vi "Experiment header-Interface module.vi"(4 "Value to change":variant, 6 "Name of parameter to update":string, 7 "Header file sections":T21=enum."GLOBAL PARAMETERS", 8 "error in (no error)":errorcluster, 9 "All header parameters in":T1={"LOGIN"={"User"="Olympus  20X", "Profile"="", "Software Version"="", "Experiment Date Time"=timestamp(0 s since 1904-01-01)}, "GLOBAL PARAMETERS"={"MicroscopeID"="", "Microscope Type"="", "Objective"="", "Field of View (um)"=0.0, "Fill time (us)"=0.0, "Experiment Type"=enum."In vivo", "Stimuli Trigger"=FALSE, "Speed Logging"=FALSE}, "IMAGING MODES"={"Time Series"=FALSE, "Motor Zstack"=FALSE, "AOL Zstack"=FALSE, "Functional Imaging"=FALSE, "Volume Imaging"=FALSE}, "TIME SERIES"={"Basic Image meta data"={"Wavelength (nm)"=0.0, "# averaged frames"=0.0, "laser power (%)"=0.0, "Pockels"=0.0, "pixel dwell time (us)"=0.0, "pmt 1"=0.0, "pmt 2"=0.0, "back apperture"=0.0, "zoom"=0.0, "field of view"=0.0, "Frame Size"=0, "AOL x centre"=0.0, "AOL y centre"=0.0, "Stage x position"=0.0, "Stage y position"=0.0, "Stage z position"=0.0}, "AOL z"=0.0}, "MOTOR Z-STACK "={"Hdr Basic Image meta data"={"Wavelength (nm)"=0.0, "# averaged frames"=0.0, "laser power (%)"=0.0, "Pockels"=0.0, "pixel dwell time (us)"=0.0, "pmt 1"=0.0, "pmt 2"=0.0, "back apperture"=0.0, "zoom"=0.0, "field of view"=0.0, "Frame Size"=0, "AOL x centre"=0.0, "AOL y centre"=0.0, "Stage x position"=0.0, "Stage y position"=0.0, "Stage z position"=0.0}, "Z Start"=0.0, "Z Stop"=0.0, "No of Planes"=0, "Laser Power (%) at Z Start"=0.0, "Laser Power (%) at Z Stop"=0.0}, "AOL Z-STACK"={"Hdr Basic Image meta data"={"Wavelength (nm)"=0.0, "# averaged frames"=0.0, "laser power (%)"=0.0, "Pockels"=0.0, "pixel dwell time (us)"=0.0, "pmt 1"=0.0, "pmt 2"=0.0, "back apperture"=0.0, "zoom"=0.0, "field of view"=0.0, "Frame Size"=0, "AOL x centre"=0.0, "AOL y centre"=0.0, "Stage x position"=0.0, "Stage y position"=0.0, "Stage z position"=0.0}, "Z Start"=0.0, "Z Stop"=0.0, "No of Planes"=0, "Laser Power (%) at Z Start"=0.0, "Laser Power (%) at Z Stop"=0.0}, "FUNCTIONAL IMAGING"={"Functional Mode"=enum."Point", "Variable Length"=FALSE, "Variable Resolution"=FALSE, "Pockels Modulation"=FALSE, "Stimuli Trigger"=FALSE, "Cool down enabled"=FALSE, "AOL Mode"=enum."Raster", "Plane Mode"=0, "Miniscan Dwell time per pixel (us)"=0.0, "poi dwell time"=0.0, "Number of trials"=0.0, "Number of cycles"=0.0, "Number of pois"=0.0, "Number of miniscans"=0.0, "Number of pixels in miniscan"=0.0, "Rectangle ROI length"=0.0, "Rectangle ROI height"=0.0, "Frame rate (fps)"=0.0, "Acquisition Length"=0.0, "video length (sec)"=0.0, "Stimuli delay (sec)"=0.0, "Cool down time (sec)"=0.0, "Basic Image meta data"={"Wavelength (nm)"=0.0, "# averaged frames"=0.0, "laser power (%)"=0.0, "Pockels"=0.0, "pixel dwell time (us)"=0.0, "pmt 1"=0.0, "pmt 2"=0.0, "back apperture"=0.0, "zoom"=0.0, "field of view"=0.0, "Frame Size"=0, "AOL x centre"=0.0, "AOL y centre"=0.0, "Stage x position"=0.0, "Stage y position"=0.0, "Stage z position"=0.0}, "Z Start (um)"=0.0, "Z Stop (um)"=0.0}, "VOLUME IMAGING"={"Functional Mode"=enum."Point", "Variable Length"=FALSE, "Variable Resolution"=FALSE, "Pockels Modulation"=FALSE, "Stimuli Trigger"=FALSE, "Cool down enabled"=FALSE, "AOL Mode"=enum."Raster", "Plane Mode"=0, "Miniscan Dwell time per pixel (us)"=0.0, "poi dwell time"=0.0, "Number of trials"=0.0, "Number of cycles"=0.0, "Number of pois"=0.0, "Number of miniscans"=0.0, "Number of pixels in miniscan"=0.0, "Rectangle ROI length"=0.0, "Rectangle ROI height"=0.0, "Frame rate (fps)"=0.0, "Acquisition Length"=0.0, "video length (sec)"=0.0, "Stimuli delay (sec)"=0.0, "Cool down time (sec)"=0.0, "Basic Image meta data"={"Wavelength (nm)"=0.0, "# averaged frames"=0.0, "laser power (%)"=0.0, "Pockels"=0.0, "pixel dwell time (us)"=0.0, "pmt 1"=0.0, "pmt 2"=0.0, "back apperture"=0.0, "zoom"=0.0, "field of view"=0.0, "Frame Size"=0, "AOL x centre"=0.0, "AOL y centre"=0.0, "Stage x position"=0.0, "Stage y position"=0.0, "Stage z position"=0.0}, "Z Start (um)"=0.0, "Z Stop (um)"=0.0}, "MOVEMENT CORRECTION"={"Movement Correction"=FALSE, "Axial Reference"=FALSE, "Reference Source"=enum."Green channel", "Full Frame Size"=0.0, "Reference Field of View"=0.0, "Reference Zoom"=0.0, "Reference dwell time (us)"=0.0, "Reference X Pixels"=0.0, "Reference Y Pixels"=0.0, "Number of Z lines"=0.0, "Size of Z pixels"=0.0, "Axial Pixels"=0.0, "Ignore Z lines"=0.0, "Reference Scan Cycles"=0.0, "Reference Threshold XY"=0.0, "Reference Threshold Z"=0.0, "Reference Average XY"=0.0, "Reference Average Z"=0.0, "Proportional Scale"=0.0, "Integral Scale"=0.0, "Proportional Scale Z"=0.0, "Integral Scale Z"=0.0, "Diff Threshold"=0.0, "Diff Threshold Z"=0.0, "Sliding Average"=FALSE, "Reference count reset enabled"=FALSE, "Scan Interval (ms)"=0.0, "Ref Plot Refresh Rate (ms)"=0.0}, "CALIBRATION"={"Pockels Calibration File"=path "", "Calibration_ini file"=path "", "Setup_ini file"=path ""}, "STATISTICS"={"Z-stack duration (sec)"=0.0, "Number of acquired data-points"=0.0, "Acquisition time (ms)"=0.0, "Number of acquired frames"=0.0, "Intertrial times"=[]}, "BIOLOGY INFORMATION"={"Animal Code or Name"="", "Animal DoB"="", "Animal Age"="", "Animal Sex"="", "Animal Weight"="", "Date of Injection"="", "Date of Implant"="", "Site of Injection"="", "Animal Ear Notch"="", "AAV constructs"="", "Genetic background"="", "Optical reporter"="", "Region of brain imaged"="", "Other \ncomments"=""}, "Calibration Data"={"Objective Name"="", "Calibration Wavelength"=0.0, "Sum X"=0.0, "Sum Y"=0.0, "Diff X"=0.0, "Diff Y"=0.0, "Distortion Correction"=0.0, " Z norm to um Scaling"=0.0, " X norm to um Scaling"=0.0}} {"VOLUME IMAGING"."Plane Mode" items=["XY Plane", "XZ Plane", "YZ Plane", "arbitraryplane"]; "VOLUME IMAGING"."Basic Image meta data"."Frame Size" items=["100X100"=100, "128X128"=128, "200X200"=200, "256X256"=256, "512X512"=512, "1024x1024"=1024, "2048x2048"=2048]; "AOL Z-STACK"."Hdr Basic Image meta data"."Frame Size" items=["100X100"=100, "128X128"=128, "200X200"=200, "256X256"=256, "512X512"=512, "1024x1024"=1024, "2048x2048"=2048]; "MOTOR Z-STACK"."Hdr Basic Image meta data"."Frame Size" items=["100X100"=100, "128X128"=128, "200X200"=200, "256X256"=256, "512X512"=512, "1024x1024"=1024, "2048x2048"=2048]; "FUNCTIONAL IMAGING"."Plane Mode" items=["XY Plane", "XZ Plane", "YZ Plane", "arbitraryplane"]; "FUNCTIONAL IMAGING"."Basic Image meta data"."Frame Size" items=["100X100"=100, "128X128"=128, "200X200"=200, "256X256"=256, "512X512"=512, "1024x1024"=1024, "2048x2048"=2048]; "TIME SERIES"."Basic Image meta data"."Frame Size" items=["100X100"=100, "128X128"=128, "200X200"=200, "256X256"=256, "512X512"=512, "1024x1024"=1024, "2048x2048"=2048]}, 10 "Function":T22, 11 "Experiment data folder path":path) -> (0 "error out":errorcluster, 1 "All params (internal)":T1 {"VOLUME IMAGING"."Plane Mode" items=["XY Plane", "XZ Plane", "YZ Plane", "arbitraryplane"]; "VOLUME IMAGING"."Basic Image meta data"."Frame Size" items=["100X100"=100, "128X128"=128, "200X200"=200, "256X256"=256, "512X512"=512, "1024x1024"=1024, "2048x2048"=2048]; "AOL Z-STACK"."Hdr Basic Image meta data"."Frame Size" items=["100X100"=100, "128X128"=128, "200X200"=200, "256X256"=256, "512X512"=512, "1024x1024"=1024, "2048x2048"=2048]; "MOTOR Z-STACK"."Hdr Basic Image meta data"."Frame Size" items=["100X100"=100, "128X128"=128, "200X200"=200, "256X256"=256, "512X512"=512, "1024x1024"=1024, "2048x2048"=2048]; "FUNCTIONAL IMAGING"."Plane Mode" items=["XY Plane", "XZ Plane", "YZ Plane", "arbitraryplane"]; "FUNCTIONAL IMAGING"."Basic Image meta data"."Frame Size" items=["100X100"=100, "128X128"=128, "200X200"=200, "256X256"=256, "512X512"=512, "1024x1024"=1024, "2048x2048"=2048]; "TIME SERIES"."Basic Image meta data"."Frame Size" items=["100X100"=100, "128X128"=128, "200X200"=200, "256X256"=256, "512X512"=512, "1024x1024"=1024, "2048x2048"=2048]})   [LabVIEW 2020]
uses:
  Typedefs/Header file interface module functions enum.ctl
  Typedefs/Header parameters cluster-ALL.ctl
  Typedefs/Header subclusters/Header params -Login.ctl
  Typedefs/Header subclusters/Header params-Global Parameters.ctl
  Misc/Experiment Type.ctl
  Typedefs/Header subclusters/Header params-Imaging Modes.ctl
  Typedefs/Header subclusters/Header params-Time Series.ctl
  Typedefs/Header subclusters/Header params-Basic image meta data.ctl
  Typedefs/Frame Size.ctl
  Typedefs/Header subclusters/Header params-Motor Z-stack.ctl
  Typedefs/Header subclusters/Header params-AOL Z-stack.ctl
  Typedefs/Header subclusters/Header params-Functional Imaging.ctl
  Typedefs/Functional Mode.ctl
  Typedefs/AOL modes.ctl
  Typedefs/Plane Mode.ctl
  Typedefs/Header subclusters/Header params-Movement correction.ctl
  Typedefs/Reference source.ctl
  Typedefs/Header subclusters/Header params-Calibration Setup.ctl
  Typedefs/Header subclusters/Header params-statistics.ctl
  Misc/Biology Information.ctl
  Typedefs/Header subclusters/Header params-calibration data.ctl
  Typedefs/Header file sections.ctl
  Typedefs/Header file actions.ctl
  Typedefs/Save-Load-Save as-Load last enum.ctl
panel:
  in  "All params (internal)":T1={"LOGIN"={"User"="Olympus  20X", "Profile"="", "Software Version"="", "Experiment Date Time"=timestamp(0 s since 1904-01-01)}, "GLOBAL PARAMETERS"={"MicroscopeID"="", "Microscope Type"="", "Objective"="", "Field of View (um)"=0.0, "Fill time (us)"=0.0, "Experiment Type"=enum."In vivo", "Stimuli Trigger"=FALSE, "Speed Logging"=FALSE}, "IMAGING MODES"={"Time Series"=FALSE, "Motor Zstack"=FALSE, "AOL Zstack"=FALSE, "Functional Imaging"=FALSE, "Volume Imaging"=FALSE}, "TIME SERIES"={"Basic Image meta data"={"Wavelength (nm)"=0.0, "# averaged frames"=0.0, "laser power (%)"=0.0, "Pockels"=0.0, "pixel dwell time (us)"=0.0, "pmt 1"=0.0, "pmt 2"=0.0, "back apperture"=0.0, "zoom"=0.0, "field of view"=0.0, "Frame Size"=0, "AOL x centre"=0.0, "AOL y centre"=0.0, "Stage x position"=0.0, "Stage y position"=0.0, "Stage z position"=0.0}, "AOL z"=0.0}, "MOTOR Z-STACK "={"Hdr Basic Image meta data"={"Wavelength (nm)"=0.0, "# averaged frames"=0.0, "laser power (%)"=0.0, "Pockels"=0.0, "pixel dwell time (us)"=0.0, "pmt 1"=0.0, "pmt 2"=0.0, "back apperture"=0.0, "zoom"=0.0, "field of view"=0.0, "Frame Size"=0, "AOL x centre"=0.0, "AOL y centre"=0.0, "Stage x position"=0.0, "Stage y position"=0.0, "Stage z position"=0.0}, "Z Start"=0.0, "Z Stop"=0.0, "No of Planes"=0, "Laser Power (%) at Z Start"=0.0, "Laser Power (%) at Z Stop"=0.0}, "AOL Z-STACK"={"Hdr Basic Image meta data"={"Wavelength (nm)"=0.0, "# averaged frames"=0.0, "laser power (%)"=0.0, "Pockels"=0.0, "pixel dwell time (us)"=0.0, "pmt 1"=0.0, "pmt 2"=0.0, "back apperture"=0.0, "zoom"=0.0, "field of view"=0.0, "Frame Size"=0, "AOL x centre"=0.0, "AOL y centre"=0.0, "Stage x position"=0.0, "Stage y position"=0.0, "Stage z position"=0.0}, "Z Start"=0.0, "Z Stop"=0.0, "No of Planes"=0, "Laser Power (%) at Z Start"=0.0, "Laser Power (%) at Z Stop"=0.0}, "FUNCTIONAL IMAGING"={"Functional Mode"=enum."Point", "Variable Length"=FALSE, "Variable Resolution"=FALSE, "Pockels Modulation"=FALSE, "Stimuli Trigger"=FALSE, "Cool down enabled"=FALSE, "AOL Mode"=enum."Raster", "Plane Mode"=0, "Miniscan Dwell time per pixel (us)"=0.0, "poi dwell time"=0.0, "Number of trials"=0.0, "Number of cycles"=0.0, "Number of pois"=0.0, "Number of miniscans"=0.0, "Number of pixels in miniscan"=0.0, "Rectangle ROI length"=0.0, "Rectangle ROI height"=0.0, "Frame rate (fps)"=0.0, "Acquisition Length"=0.0, "video length (sec)"=0.0, "Stimuli delay (sec)"=0.0, "Cool down time (sec)"=0.0, "Basic Image meta data"={"Wavelength (nm)"=0.0, "# averaged frames"=0.0, "laser power (%)"=0.0, "Pockels"=0.0, "pixel dwell time (us)"=0.0, "pmt 1"=0.0, "pmt 2"=0.0, "back apperture"=0.0, "zoom"=0.0, "field of view"=0.0, "Frame Size"=0, "AOL x centre"=0.0, "AOL y centre"=0.0, "Stage x position"=0.0, "Stage y position"=0.0, "Stage z position"=0.0}, "Z Start (um)"=0.0, "Z Stop (um)"=0.0}, "VOLUME IMAGING"={"Functional Mode"=enum."Point", "Variable Length"=FALSE, "Variable Resolution"=FALSE, "Pockels Modulation"=FALSE, "Stimuli Trigger"=FALSE, "Cool down enabled"=FALSE, "AOL Mode"=enum."Raster", "Plane Mode"=0, "Miniscan Dwell time per pixel (us)"=0.0, "poi dwell time"=0.0, "Number of trials"=0.0, "Number of cycles"=0.0, "Number of pois"=0.0, "Number of miniscans"=0.0, "Number of pixels in miniscan"=0.0, "Rectangle ROI length"=0.0, "Rectangle ROI height"=0.0, "Frame rate (fps)"=0.0, "Acquisition Length"=0.0, "video length (sec)"=0.0, "Stimuli delay (sec)"=0.0, "Cool down time (sec)"=0.0, "Basic Image meta data"={"Wavelength (nm)"=0.0, "# averaged frames"=0.0, "laser power (%)"=0.0, "Pockels"=0.0, "pixel dwell time (us)"=0.0, "pmt 1"=0.0, "pmt 2"=0.0, "back apperture"=0.0, "zoom"=0.0, "field of view"=0.0, "Frame Size"=0, "AOL x centre"=0.0, "AOL y centre"=0.0, "Stage x position"=0.0, "Stage y position"=0.0, "Stage z position"=0.0}, "Z Start (um)"=0.0, "Z Stop (um)"=0.0}, "MOVEMENT CORRECTION"={"Movement Correction"=FALSE, "Axial Reference"=FALSE, "Reference Source"=enum."Green channel", "Full Frame Size"=0.0, "Reference Field of View"=0.0, "Reference Zoom"=0.0, "Reference dwell time (us)"=0.0, "Reference X Pixels"=0.0, "Reference Y Pixels"=0.0, "Number of Z lines"=0.0, "Size of Z pixels"=0.0, "Axial Pixels"=0.0, "Ignore Z lines"=0.0, "Reference Scan Cycles"=0.0, "Reference Threshold XY"=0.0, "Reference Threshold Z"=0.0, "Reference Average XY"=0.0, "Reference Average Z"=0.0, "Proportional Scale"=0.0, "Integral Scale"=0.0, "Proportional Scale Z"=0.0, "Integral Scale Z"=0.0, "Diff Threshold"=0.0, "Diff Threshold Z"=0.0, "Sliding Average"=FALSE, "Reference count reset enabled"=FALSE, "Scan Interval (ms)"=0.0, "Ref Plot Refresh Rate (ms)"=0.0}, "CALIBRATION"={"Pockels Calibration File"=path "", "Calibration_ini file"=path "", "Setup_ini file"=path ""}, "STATISTICS"={"Z-stack duration (sec)"=0.0, "Number of acquired data-points"=0.0, "Acquisition time (ms)"=0.0, "Number of acquired frames"=0.0, "Intertrial times"=[]}, "BIOLOGY INFORMATION"={"Animal Code or Name"="", "Animal DoB"="", "Animal Age"="", "Animal Sex"="", "Animal Weight"="", "Date of Injection"="", "Date of Implant"="", "Site of Injection"="", "Animal Ear Notch"="", "AAV constructs"="", "Genetic background"="", "Optical reporter"="", "Region of brain imaged"="", "Other \ncomments"=""}, "Calibration Data"={"Objective Name"="", "Calibration Wavelength"=0.0, "Sum X"=0.0, "Sum Y"=0.0, "Diff X"=0.0, "Diff Y"=0.0, "Distortion Correction"=0.0, " Z norm to um Scaling"=0.0, " X norm to um Scaling"=0.0}} {"VOLUME IMAGING"."Plane Mode" items=["XY Plane", "XZ Plane", "YZ Plane", "arbitraryplane"]; "VOLUME IMAGING"."Basic Image meta data"."Frame Size" items=["100X100"=100, "128X128"=128, "200X200"=200, "256X256"=256, "512X512"=512, "1024x1024"=1024, "2048x2048"=2048]; "AOL Z-STACK"."Hdr Basic Image meta data"."Frame Size" items=["100X100"=100, "128X128"=128, "200X200"=200, "256X256"=256, "512X512"=512, "1024x1024"=1024, "2048x2048"=2048]; "MOTOR Z-STACK"."Hdr Basic Image meta data"."Frame Size" items=["100X100"=100, "128X128"=128, "200X200"=200, "256X256"=256, "512X512"=512, "1024x1024"=1024, "2048x2048"=2048]; "FUNCTIONAL IMAGING"."Plane Mode" items=["XY Plane", "XZ Plane", "YZ Plane", "arbitraryplane"]; "FUNCTIONAL IMAGING"."Basic Image meta data"."Frame Size" items=["100X100"=100, "128X128"=128, "200X200"=200, "256X256"=256, "512X512"=512, "1024x1024"=1024, "2048x2048"=2048]; "TIME SERIES"."Basic Image meta data"."Frame Size" items=["100X100"=100, "128X128"=128, "200X200"=200, "256X256"=256, "512X512"=512, "1024x1024"=1024, "2048x2048"=2048]}
  # "Used with the \"Update specific value in memory\" function only"
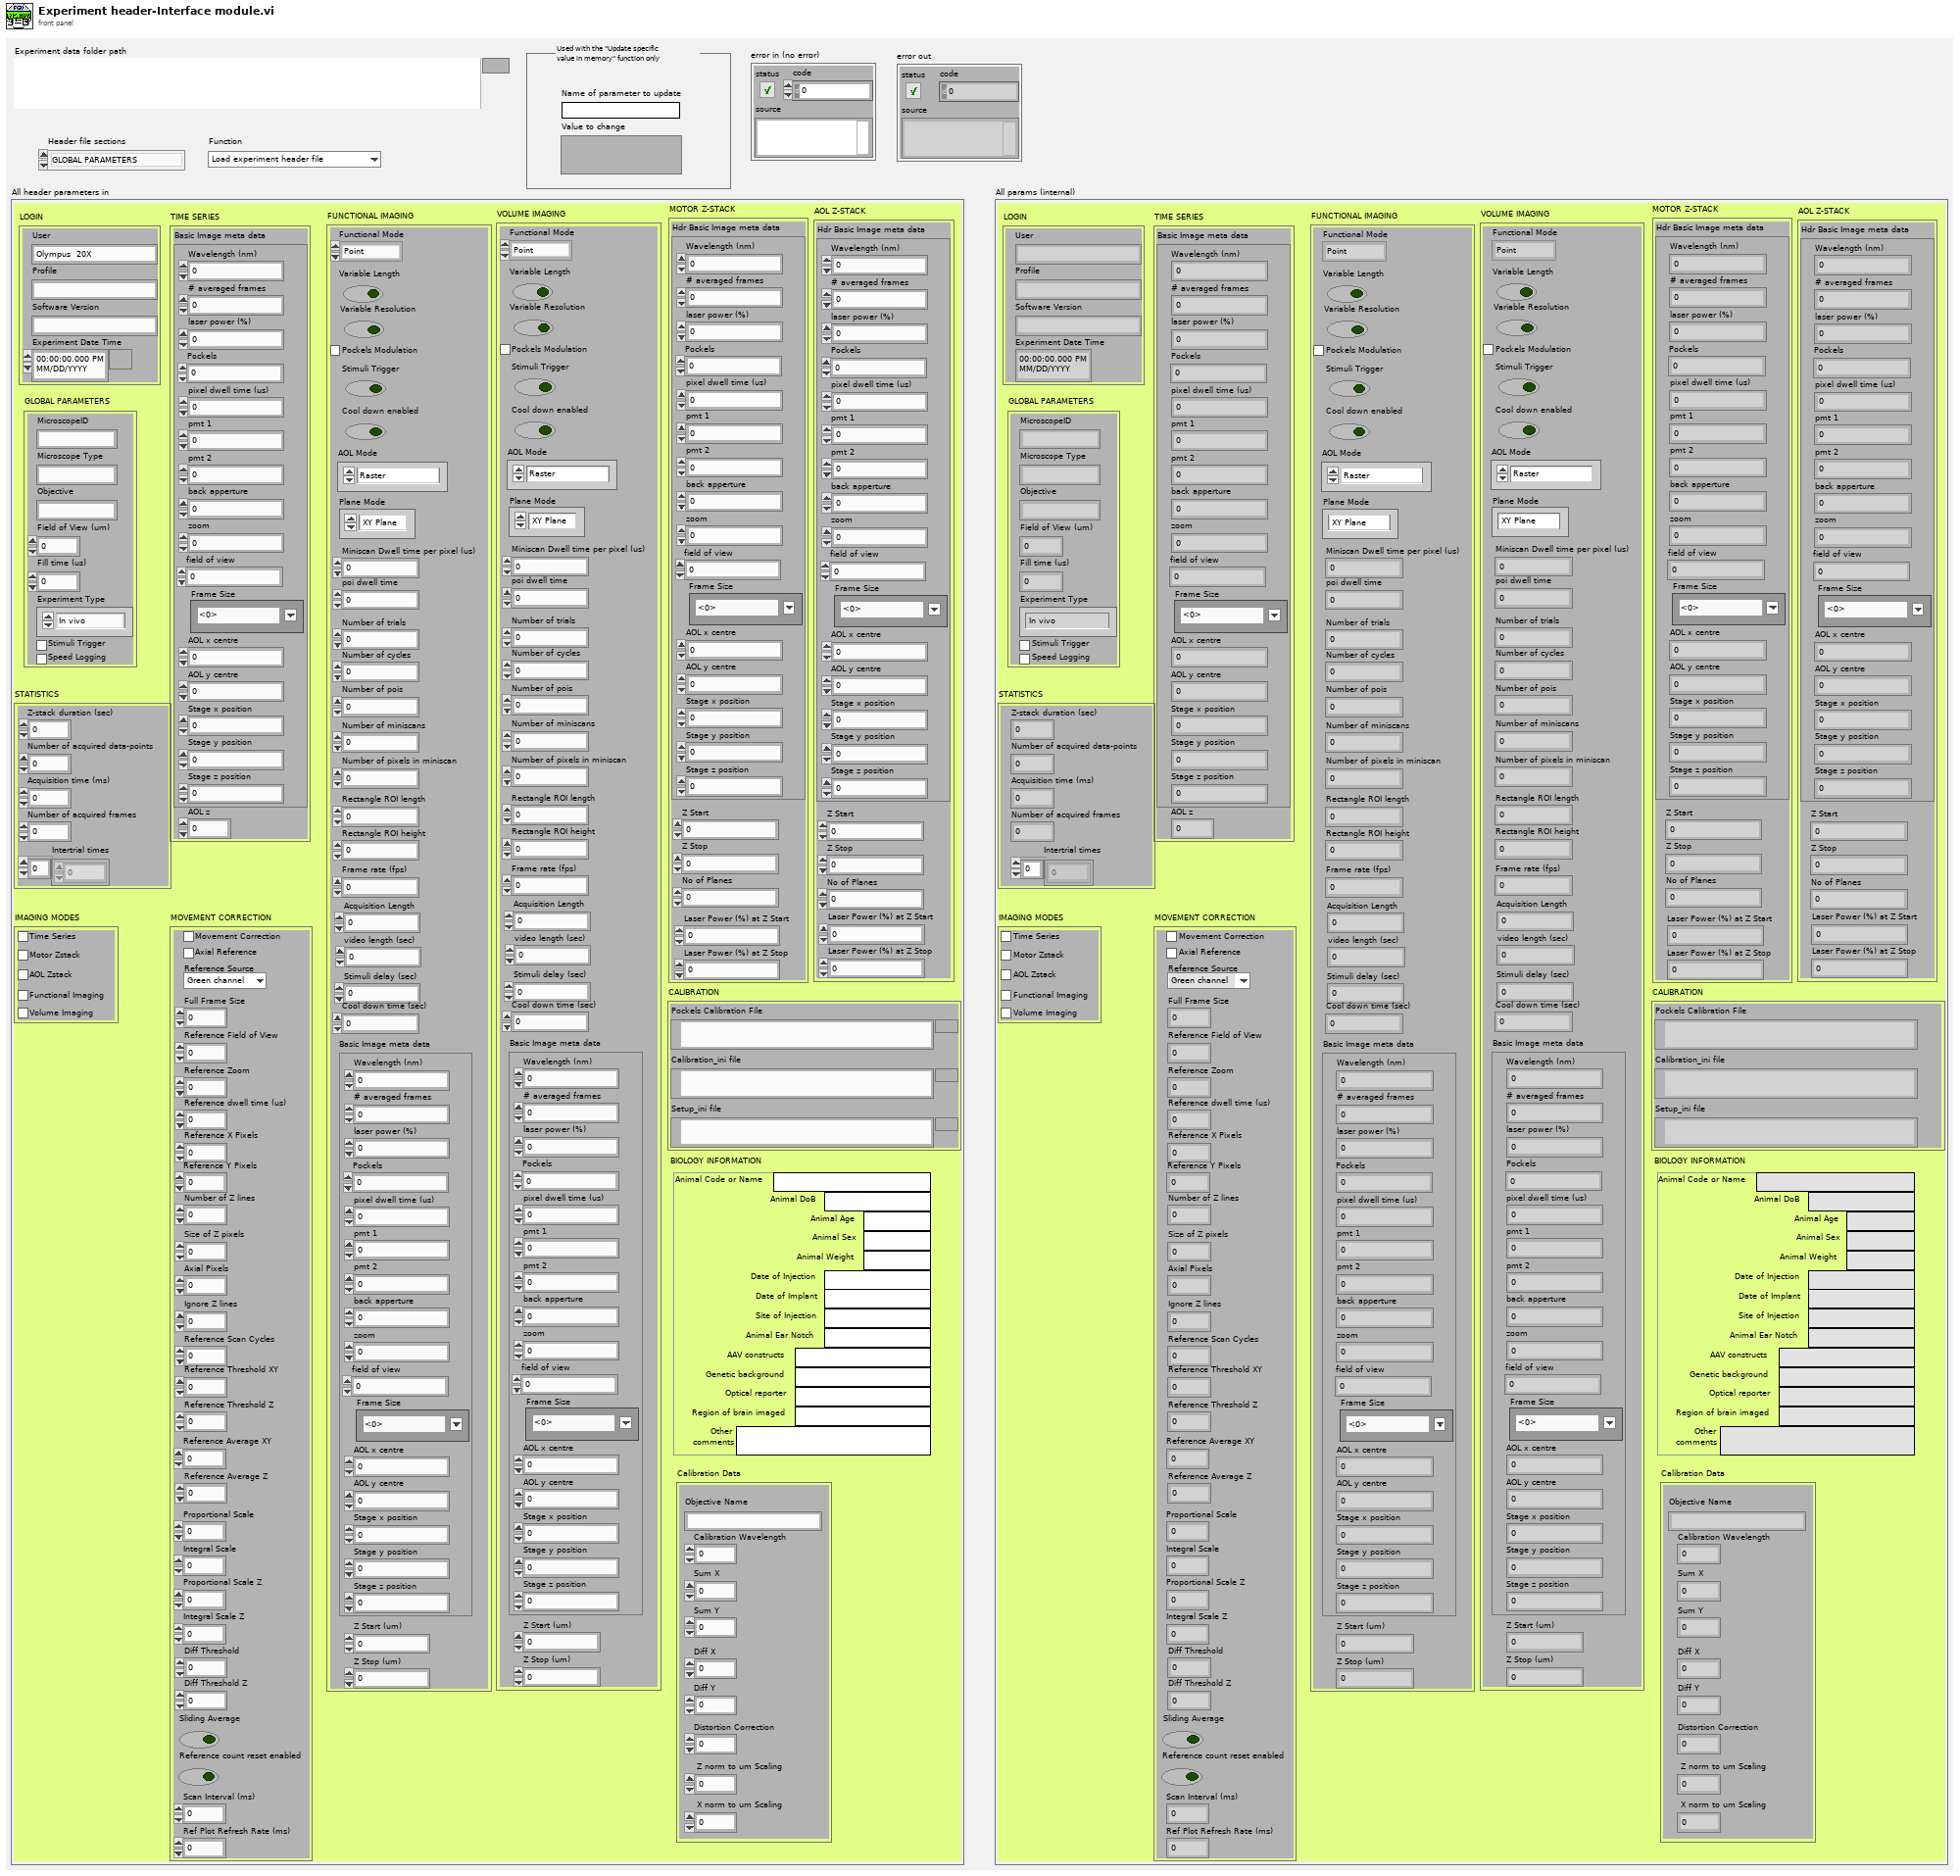
[diagram p1: front panel]
types:
  T1 = typedef "Header parameters cluster-ALL.ctl" = cluster{"LOGIN":T2, "GLOBAL PARAMETERS":T3, "IMAGING MODES":T5, "TIME SERIES":T6, "MOTOR Z-STACK ":T9, "AOL Z-STACK":T10, "FUNCTIONAL IMAGING":T11, "VOLUME IMAGING":T11, "MOVEMENT CORRECTION":T15, "CALIBRATION":T17, "STATISTICS":T18, "BIOLOGY INFORMATION":T19, "Calibration Data":T20}
  T2 = typedef "Header params -Login.ctl" = cluster{"User":string, "Profile":string, "Software Version":string, "Experiment Date Time":timestamp}
  T3 = typedef "Header params-Global Parameters.ctl" = cluster{"MicroscopeID":string, "Microscope Type":string, "Objective":string, "Field of View (um)":dbl, "Fill time (us)":dbl, "Experiment Type":T4, "Stimuli Trigger":bool, "Speed Logging":bool}
  T4 = typedef "Experiment Type.ctl" = enum16{"In vivo", "In vitro", "Testing", "Calibration", "Other"}
  T5 = typedef "Header params-Imaging Modes.ctl" = cluster{"Time Series":bool, "Motor Zstack":bool, "AOL Zstack":bool, "Functional Imaging":bool, "Volume Imaging":bool}
  T6 = typedef "Header params-Time Series.ctl" = cluster{"Basic Image meta data":T7, "AOL z":dbl}
  T7 = typedef "Header params-Basic image meta data.ctl" = cluster{"Wavelength (nm)":dbl, "# averaged frames":dbl, "laser power (%)":dbl, "Pockels":dbl, "pixel dwell time (us)":dbl, "pmt 1":dbl, "pmt 2":dbl, "back apperture":dbl, "zoom":dbl, "field of view":dbl, "Frame Size":T8, "AOL x centre":dbl, "AOL y centre":dbl, "Stage x position":dbl, "Stage y position":dbl, "Stage z position":dbl}
  T8 = typedef "Frame Size.ctl" = u16
  T9 = typedef "Header params-Motor Z-stack.ctl" = cluster{"Hdr Basic Image meta data":T7, "Z Start":dbl, "Z Stop":dbl, "No of Planes":i32, "Laser Power (%) at Z Start":dbl, "Laser Power (%) at Z Stop":dbl}
  T10 = typedef "Header params-AOL Z-stack.ctl" = cluster{"Hdr Basic Image meta data":T7, "Z Start":dbl, "Z Stop":dbl, "No of Planes":i32, "Laser Power (%) at Z Start":dbl, "Laser Power (%) at Z Stop":dbl}
  T11 = typedef "Header params-Functional Imaging.ctl" = cluster{"Functional Mode":T12, "Variable Length":bool, "Variable Resolution":bool, "Pockels Modulation":bool, "Stimuli Trigger":bool, "Cool down enabled":bool, "AOL Mode":T13, "Plane Mode":T14, "Miniscan Dwell time per pixel (us)":dbl, "poi dwell time":dbl, "Number of trials":dbl, "Number of cycles":dbl, "Number of pois":dbl, "Number of miniscans":dbl, "Number of pixels in miniscan":dbl, "Rectangle ROI length":dbl, "Rectangle ROI height":dbl, "Frame rate (fps)":dbl, "Acquisition Length":dbl, "video length (sec)":dbl, "Stimuli delay (sec)":dbl, "Cool down time (sec)":dbl, "Basic Image meta data":T7, "Z Start (um)":dbl, "Z Stop (um)":dbl}
  T12 = typedef "Functional Mode.ctl" = enum16{"Point", "Line", "Patch", "Plane", "Volume"}
  T13 = typedef "AOL modes.ctl" = enum16{"Raster", "Structural", "Pointing", "Mini Scan", "Alignment"}
  T14 = typedef "Plane Mode.ctl" = u16
  T15 = typedef "Header params-Movement correction.ctl" = cluster{"Movement Correction":bool, "Axial Reference":bool, "Reference Source":T16, "Full Frame Size":dbl, "Reference Field of View":dbl, "Reference Zoom":dbl, "Reference dwell time (us)":dbl, "Reference X Pixels":dbl, "Reference Y Pixels":dbl, "Number of Z lines":dbl, "Size of Z pixels":dbl, "Axial Pixels":dbl, "Ignore Z lines":dbl, "Reference Scan Cycles":dbl, "Reference Threshold XY":dbl, "Reference Threshold Z":dbl, "Reference Average XY":dbl, "Reference Average Z":dbl, "Proportional Scale":dbl, "Integral Scale":dbl, "Proportional Scale Z":dbl, "Integral Scale Z":dbl, "Diff Threshold":dbl, "Diff Threshold Z":dbl, "Sliding Average":bool, "Reference count reset enabled":bool, "Scan Interval (ms)":dbl, "Ref Plot Refresh Rate (ms)":dbl}
  T16 = typedef "Reference source.ctl" = enum16{"Green channel", "Red channel"}
  T17 = typedef "Header params-Calibration Setup.ctl" = cluster{"Pockels Calibration File":path, "Calibration_ini file":path, "Setup_ini file":path}
  T18 = typedef "Header params-statistics.ctl" = cluster{"Z-stack duration (sec)":dbl, "Number of acquired data-points":dbl, "Acquisition time (ms)":dbl, "Number of acquired frames":dbl, "Intertrial times":dbl[]}
  T19 = typedef "Biology Information.ctl" = cluster{"Animal Code or Name":string, "Animal DoB":string, "Animal Age":string, "Animal Sex":string, "Animal Weight":string, "Date of Injection":string, "Date of Implant":string, "Site of Injection":string, "Animal Ear Notch":string, "AAV constructs":string, "Genetic background":string, "Optical reporter":string, "Region of brain imaged":string, "Other \ncomments":string}
  T20 = typedef "Header params-calibration data.ctl" = cluster{"Objective Name":string, "Calibration Wavelength":dbl, "Sum X":dbl, "Sum Y":dbl, "Diff X":dbl, "Diff Y":dbl, "Distortion Correction":dbl, " Z norm to um Scaling":dbl, " X norm to um Scaling":dbl}
  T21 = typedef "Header file sections.ctl" = enum16{"ALL SECTIONS", "LOGIN", "GLOBAL PARAMETERS", "CALIBRATION DATA", "IMAGING MODES", "TIME SERIES", "MOTOR Z-STACK", "AOL Z-STACK", "FUNCTIONAL IMAGING", "VOLUME IMAGING", "MOVEMENT CORRECTION", "CALIBRATION", "STATISTICS", "BIOLOGY INFORMATION"}
  T22 = typedef "Header file interface module functions enum.ctl" = enum16{"Load experiment header file", "Save experiment header file", "Clear stored values", "Read stored values", "Update specific value in memory", "Update values in memory"}
  T23 = typedef "Header file actions.ctl" = enum16{"Create", "Open", "Read All", "Read Section", "Write All", "Write Section", "Close"}
  T24 = typedef "Save-Load-Save as-Load last enum.ctl" = enum16{"Save file", "Save file as", "Load file", "Load last file"}
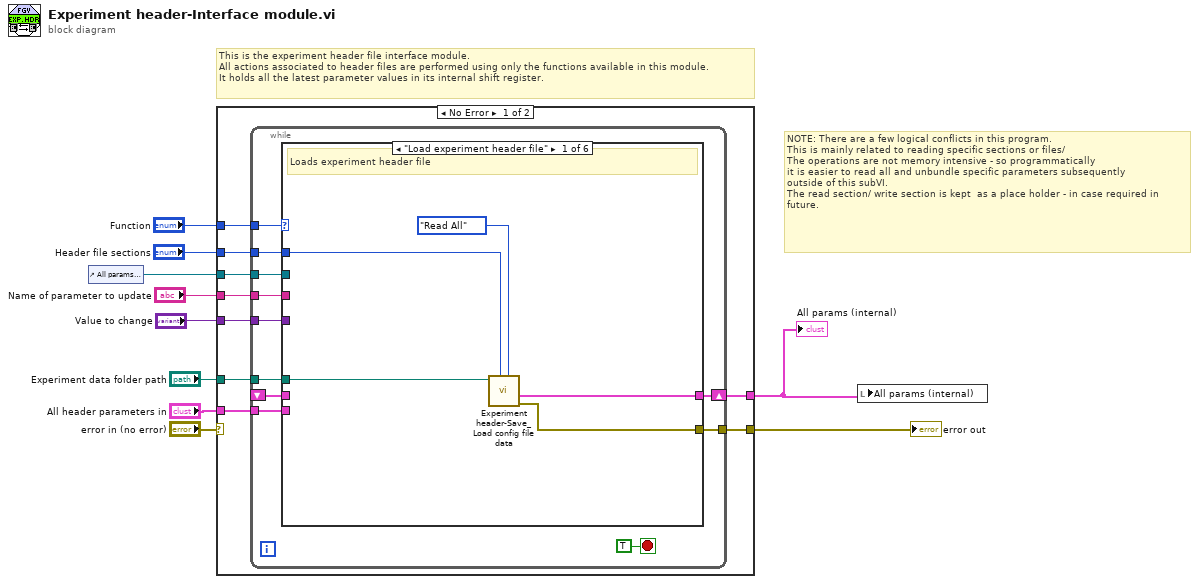
[diagram p0: block diagram]
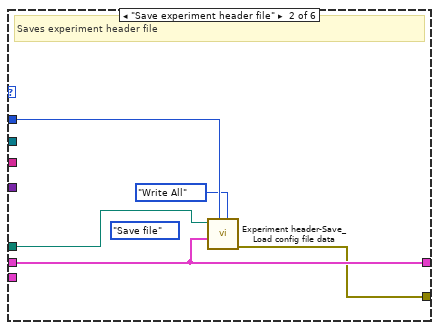
[diagram p2: hidden frame]
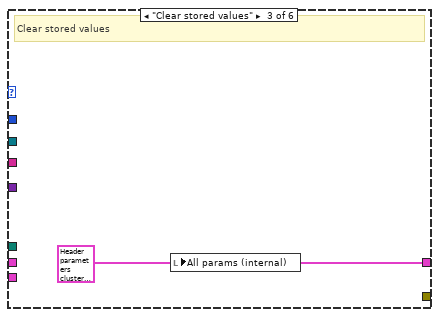
[diagram p3: hidden frame]
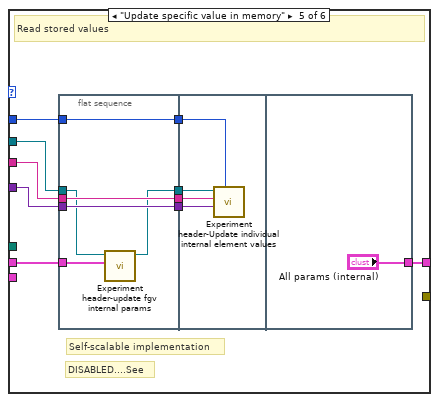
[diagram p5: hidden frame]
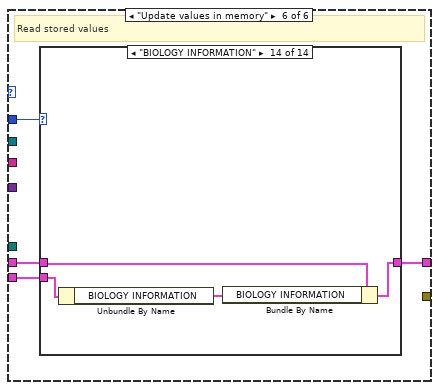
[diagram p6: hidden frame]
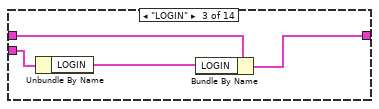
[diagram p9: hidden frame]
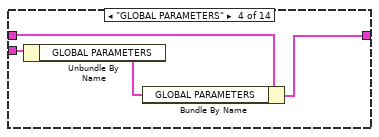
[diagram p10: hidden frame]
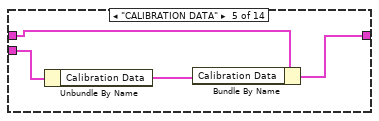
[diagram p11: hidden frame]
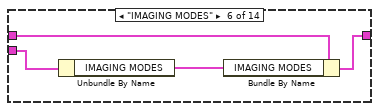
[diagram p12: hidden frame]
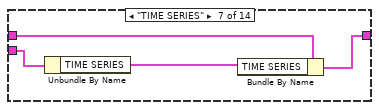
[diagram p13: hidden frame]
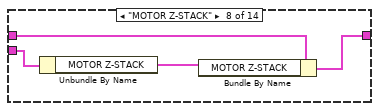
[diagram p14: hidden frame]
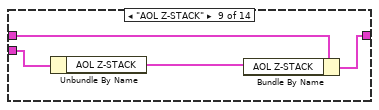
[diagram p15: hidden frame]
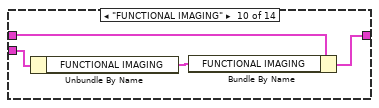
[diagram p16: hidden frame]
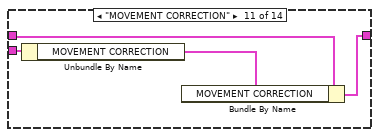
[diagram p17: hidden frame]
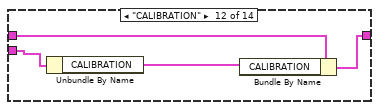
[diagram p18: hidden frame]
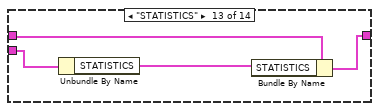
[diagram p19: hidden frame]
diagram:
  # "NOTE: There are a few logical conflicts in this program.\nThis is mainly related to reading specific sections or files/\nThe operations are not memory intensive - so programmatically\nit is easier to read all and unbundle specific parameters subsequently\noutside of this subVI.\nThe read section/ write section is kept  as a place holder - in case required in \nfuture."
  # "This is the experiment header file interface module.\nAll actions associated to header files are performed using only the functions available in this module.\nIt holds all the latest parameter values in its internal shift register."
  n1 = control-ref of="All params (internal)"() -> (w1:refnum<vi>)
  n2 = case shown="No Error" "error in (no error)" {
    selector: "error in (no error)" -> [_ w118]
    tunnel: [w19 _] -> w2
    tunnel: "Function" -> [w18 _]
    tunnel: "Name of parameter to update" -> [w17 _]
    tunnel: "Value to change" -> [w16 _]
    tunnel: "Experiment data folder path" -> [w15 _]
    tunnel: [w14 w118] -> w8
    tunnel: "All header parameters in" -> [w13 _]
    tunnel: "Header file sections" -> [w12 _]
    tunnel: w1 -> [w11 _]
    frame No Error {
      n3 = while {
        shift-right: [w29] -> w19
        shift-left: _ -> [w27]
        tunnel: w18 -> [w28]
        tunnel: w17 -> [w26]
        tunnel: w16 -> [w25]
        tunnel: w15 -> [w23]
        tunnel: [w24] -> w14
        tunnel: w13 -> [w22]
        tunnel: w12 -> [w21]
        tunnel: w11 -> [w20]
        stop <- TRUE stop-if-true
        n4 = case shown="\"Load experiment header file\"" w28 {
          tunnel: [w32 w39 w41 w42 w50 w65] -> w29
          tunnel: w27 -> [_ w39 _ w42 w43 w64]
          tunnel: w26 -> [_ _ _ _ w52 _]
          tunnel: w25 -> [_ _ _ _ w51 _]
          tunnel: [w34 w37 _ _ _ _] -> w24
          tunnel: w23 -> [w35 w40 _ _ _ _]
          tunnel: w22 -> [_ _ _ _ _ w66]
          tunnel: w21 -> [w33 w38 _ _ w48 w67]
          tunnel: w20 -> [_ _ _ _ w49 _]
          frame "Load experiment header file" {
            # "Loads experiment header file"
            n5 = call "Experiment header-Save_Load config file data.vi"("Header file actions"=Header_file_actions."Read All", "Header file sections"=w33, "Experiment data folder path"=w35) -> ("error out"=w34:errorcluster, "All header parameters out"=w32:T1)  [unwired: 7 in]
          }
          frame "Save experiment header file" {
            (unwired) Save-Load-Save_as-Load_last_enum."Save file" ("Function")
            # "Saves experiment header file"
            n6 = call "Experiment header-Save_Load config file data.vi"("Header file actions"=Header_file_actions."Write All", "Header file sections"=w38, "All header parameters in"=w39, "Experiment data folder path"=w40) -> ("error out"=w37:errorcluster)  [unwired: 6 in, 1 out]
          }
          frame "Clear stored values" {
            w41 = T1 {"LOGIN"={"User"="", "Profile"="", "Software Version"="", "Experiment Date Time"=timestamp(0 s since 1904-01-01)}, "GLOBAL PARAMETERS"={"MicroscopeID"="", "Microscope Type"="", "Objective"="", "Field of View (um)"=0.0, "Fill time (us)"=0.0, "Experiment Type"=enum."In vivo", "Stimuli Trigger"=FALSE, "Speed Logging"=FALSE}, "IMAGING MODES"={"Time Series"=FALSE, "Motor Zstack"=FALSE, "AOL Zstack"=FALSE, "Functional Imaging"=FALSE, "Volume Imaging"=FALSE}, "TIME SERIES"={"Basic Image meta data"={"Wavelength (nm)"=0.0, "# averaged frames"=0.0, "laser power (%)"=0.0, "Pockels"=0.0, "pixel dwell time (us)"=0.0, "pmt 1"=0.0, "pmt 2"=0.0, "back apperture"=0.0, "zoom"=0.0, "field of view"=0.0, "Frame Size"=0, "AOL x centre"=0.0, "AOL y centre"=0.0, "Stage x position"=0.0, "Stage y position"=0.0, "Stage z position"=0.0}, "AOL z"=0.0}, "MOTOR Z-STACK "={"Hdr Basic Image meta data"={"Wavelength (nm)"=0.0, "# averaged frames"=0.0, "laser power (%)"=0.0, "Pockels"=0.0, "pixel dwell time (us)"=0.0, "pmt 1"=0.0, "pmt 2"=0.0, "back apperture"=0.0, "zoom"=0.0, "field of view"=0.0, "Frame Size"=0, "AOL x centre"=0.0, "AOL y centre"=0.0, "Stage x position"=0.0, "Stage y position"=0.0, "Stage z position"=0.0}, "Z Start"=0.0, "Z Stop"=0.0, "No of Planes"=0, "Laser Power (%) at Z Start"=0.0, "Laser Power (%) at Z Stop"=0.0}, "AOL Z-STACK"={"Hdr Basic Image meta data"={"Wavelength (nm)"=0.0, "# averaged frames"=0.0, "laser power (%)"=0.0, "Pockels"=0.0, "pixel dwell time (us)"=0.0, "pmt 1"=0.0, "pmt 2"=0.0, "back apperture"=0.0, "zoom"=0.0, "field of view"=0.0, "Frame Size"=0, "AOL x centre"=0.0, "AOL y centre"=0.0, "Stage x position"=0.0, "Stage y position"=0.0, "Stage z position"=0.0}, "Z Start"=0.0, "Z Stop"=0.0, "No of Planes"=0, "Laser Power (%) at Z Start"=0.0, "Laser Power (%) at Z Stop"=0.0}, "FUNCTIONAL IMAGING"={"Functional Mode"=enum."Point", "Variable Length"=FALSE, "Variable Resolution"=FALSE, "Pockels Modulation"=FALSE, "Stimuli Trigger"=FALSE, "Cool down enabled"=FALSE, "AOL Mode"=enum."Raster", "Plane Mode"=0, "Miniscan Dwell time per pixel (us)"=0.0, "poi dwell time"=0.0, "Number of trials"=0.0, "Number of cycles"=0.0, "Number of pois"=0.0, "Number of miniscans"=0.0, "Number of pixels in miniscan"=0.0, "Rectangle ROI length"=0.0, "Rectangle ROI height"=0.0, "Frame rate (fps)"=0.0, "Acquisition Length"=0.0, "video length (sec)"=0.0, "Stimuli delay (sec)"=0.0, "Cool down time (sec)"=0.0, "Basic Image meta data"={"Wavelength (nm)"=0.0, "# averaged frames"=0.0, "laser power (%)"=0.0, "Pockels"=0.0, "pixel dwell time (us)"=0.0, "pmt 1"=0.0, "pmt 2"=0.0, "back apperture"=0.0, "zoom"=0.0, "field of view"=0.0, "Frame Size"=0, "AOL x centre"=0.0, "AOL y centre"=0.0, "Stage x position"=0.0, "Stage y position"=0.0, "Stage z position"=0.0}, "Z Start (um)"=0.0, "Z Stop (um)"=0.0}, "VOLUME IMAGING"={"Functional Mode"=enum."Point", "Variable Length"=FALSE, "Variable Resolution"=FALSE, "Pockels Modulation"=FALSE, "Stimuli Trigger"=FALSE, "Cool down enabled"=FALSE, "AOL Mode"=enum."Raster", "Plane Mode"=0, "Miniscan Dwell time per pixel (us)"=0.0, "poi dwell time"=0.0, "Number of trials"=0.0, "Number of cycles"=0.0, "Number of pois"=0.0, "Number of miniscans"=0.0, "Number of pixels in miniscan"=0.0, "Rectangle ROI length"=0.0, "Rectangle ROI height"=0.0, "Frame rate (fps)"=0.0, "Acquisition Length"=0.0, "video length (sec)"=0.0, "Stimuli delay (sec)"=0.0, "Cool down time (sec)"=0.0, "Basic Image meta data"={"Wavelength (nm)"=0.0, "# averaged frames"=0.0, "laser power (%)"=0.0, "Pockels"=0.0, "pixel dwell time (us)"=0.0, "pmt 1"=0.0, "pmt 2"=0.0, "back apperture"=0.0, "zoom"=0.0, "field of view"=0.0, "Frame Size"=0, "AOL x centre"=0.0, "AOL y centre"=0.0, "Stage x position"=0.0, "Stage y position"=0.0, "Stage z position"=0.0}, "Z Start (um)"=0.0, "Z Stop (um)"=0.0}, "MOVEMENT CORRECTION"={"Movement Correction"=FALSE, "Axial Reference"=FALSE, "Reference Source"=enum."Green channel", "Full Frame Size"=0.0, "Reference Field of View"=0.0, "Reference Zoom"=0.0, "Reference dwell time (us)"=0.0, "Reference X Pixels"=0.0, "Reference Y Pixels"=0.0, "Number of Z lines"=0.0, "Size of Z pixels"=0.0, "Axial Pixels"=0.0, "Ignore Z lines"=0.0, "Reference Scan Cycles"=0.0, "Reference Threshold XY"=0.0, "Reference Threshold Z"=0.0, "Reference Average XY"=0.0, "Reference Average Z"=0.0, "Proportional Scale"=0.0, "Integral Scale"=0.0, "Proportional Scale Z"=0.0, "Integral Scale Z"=0.0, "Diff Threshold"=0.0, "Diff Threshold Z"=0.0, "Sliding Average"=FALSE, "Reference count reset enabled"=FALSE, "Scan Interval (ms)"=0.0, "Ref Plot Refresh Rate (ms)"=0.0}, "CALIBRATION"={"Pockels Calibration File"=path "", "Calibration_ini file"=path "", "Setup_ini file"=path ""}, "STATISTICS"={"Z-stack duration (sec)"=0.0, "Number of acquired data-points"=0.0, "Acquisition time (ms)"=0.0, "Number of acquired frames"=0.0, "Intertrial times"=[]}, "BIOLOGY INFORMATION"={"Animal Code or Name"="", "Animal DoB"="", "Animal Age"="", "Animal Sex"="", "Animal Weight"="", "Date of Injection"="", "Date of Implant"="", "Site of Injection"="", "Animal Ear Notch"="", "AAV constructs"="", "Genetic background"="", "Optical reporter"="", "Region of brain imaged"="", "Other \ncomments"=""}, "Calibration Data"={"Objective Name"="", "Calibration Wavelength"=0.0, "Sum X"=0.0, "Sum Y"=0.0, "Diff X"=0.0, "Diff Y"=0.0, "Distortion Correction"=0.0, " Z norm to um Scaling"=0.0, " X norm to um Scaling"=0.0}} ("All header parameters in")
            # "Clear stored values"
            n7 = local write "All params (internal)"(w41) -> ()
          }
          frame "Read stored values", Default {
            # "Read stored values"
          }
          frame "Update specific value in memory" {
            # "DISABLED....See"
            # "Self-scalable implementation"
            # "Read stored values"
            n8 = flat-sequence {
              tunnel: w48 -> [w56]
              tunnel: w51 -> [w57]
              tunnel: w52 -> [w58]
              tunnel: w49 -> [w54]
              tunnel: [w53] -> w47
              tunnel: [w58] -> w46
              tunnel: [w57] -> w45
              tunnel: [w56] -> w44
              tunnel: w43 -> [w55]
              tunnel: w47 -> [w59]
              tunnel: w46 -> [w62]
              tunnel: w45 -> [w61]
              tunnel: w44 -> [w60]
              tunnel: ["All params (internal)"] -> w50
              frame #0 {
                n9 = call "Experiment header-update fgv internal params.vi"("All header parameters in"=w55, "All header parameters / Header module interface cluster"=w54) -> ("All header parameters OUT"=w53:refnum<vi>)  [unwired: 8 in, 1 out]
              }
              frame #1 {
                n10 = call "Experiment header-Update individual internal element values.vi"("Header file sections"=w60, "Variant"=w61, "Name of parameter to update"=w62, "All header parameters / Header module interface cluster"=w59) -> ()  [unwired: 7 in, 1 out]
              }
              frame #2 {
              }
            }
          }
          frame "Update values in memory" {
            # "Read stored values"
            n11 = case shown="\"BIOLOGY INFORMATION\"" w67 {
              tunnel: w66 -> [w68 _ w72 w74 w80 w83 w86 w91 w94 w98 w102 w106 w110 w115]
              tunnel: [w68 w69 w71 w75 w78 w82 w87 w90 w96 w100 w103 w108 w111 w114] -> w65
              tunnel: w64 -> [_ w69 w73 w76 w81 w84 w88 w92 w95 w99 w104 w107 w112 w116]
              frame "ALL SECTIONS" {
              }
              frame Default {
              }
              frame "LOGIN" {
                n12 = Unbundle By Name(w72) -> ("LOGIN"=w70:T2)
                n13 = Bundle By Name(cluster=w73, "LOGIN"=w70) -> (w71:T1)
              }
              frame "GLOBAL PARAMETERS" {
                n14 = Unbundle By Name(w74) -> ("GLOBAL PARAMETERS"=w77:T3)
                n15 = Bundle By Name(cluster=w76, "GLOBAL PARAMETERS"=w77) -> (w75:T1)
              }
              frame "CALIBRATION DATA" {
                n16 = Unbundle By Name(w80) -> ("Calibration Data"=w79:T20)
                n17 = Bundle By Name(cluster=w81, "Calibration Data"=w79) -> (w78:T1)
              }
              frame "IMAGING MODES" {
                n18 = Unbundle By Name(w83) -> ("IMAGING MODES"=w85:T5)
                n19 = Bundle By Name(cluster=w84, "IMAGING MODES"=w85) -> (w82:T1)
              }
              frame "TIME SERIES" {
                n20 = Unbundle By Name(w86) -> ("TIME SERIES"=w89:T6)
                n21 = Bundle By Name(cluster=w88, "TIME SERIES"=w89) -> (w87:T1)
              }
              frame "MOTOR Z-STACK" {
                n22 = Unbundle By Name(w91) -> ("MOTOR Z-STACK"=w93:T9)
                n23 = Bundle By Name(cluster=w92, "MOTOR Z-STACK"=w93) -> (w90:T1)
              }
              frame "AOL Z-STACK" {
                n24 = Unbundle By Name(w94) -> ("AOL Z-STACK"=w97:T10)
                n25 = Bundle By Name(cluster=w95, "AOL Z-STACK"=w97) -> (w96:T1)
              }
              frame "FUNCTIONAL IMAGING" {
                n26 = Unbundle By Name(w98) -> ("FUNCTIONAL IMAGING"=w101:T11)
                n27 = Bundle By Name(cluster=w99, "FUNCTIONAL IMAGING"=w101) -> (w100:T1)
              }
              frame "MOVEMENT CORRECTION" {
                n28 = Unbundle By Name(w102) -> ("MOVEMENT CORRECTION"=w105:T15)
                n29 = Bundle By Name(cluster=w104, "MOVEMENT CORRECTION"=w105) -> (w103:T1)
              }
              frame "CALIBRATION" {
                n30 = Unbundle By Name(w106) -> ("CALIBRATION"=w109:T17)
                n31 = Bundle By Name(cluster=w107, "CALIBRATION"=w109) -> (w108:T1)
              }
              frame "STATISTICS" {
                n32 = Unbundle By Name(w110) -> ("STATISTICS"=w113:T18)
                n33 = Bundle By Name(cluster=w112, "STATISTICS"=w113) -> (w111:T1)
              }
              frame "BIOLOGY INFORMATION" {
                n34 = Unbundle By Name(w115) -> ("BIOLOGY INFORMATION"=w117:T19)
                n35 = Bundle By Name(cluster=w116, "BIOLOGY INFORMATION"=w117) -> (w114:T1)
              }
            }
          }
        }
      }
    }
    frame Error {
    }
  }
  "error out" <- w8
  "All params (internal)" <- w2
  n36 = local write "All params (internal)"(w2) -> ()
